vi "Test1.vi"() -> ()   [LabVIEW 2015]
panel:
  out "数值":i32
  in  "停止":bool
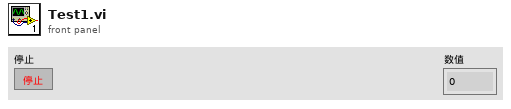
[diagram p1: front panel]
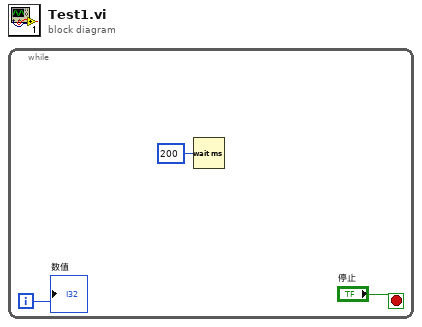
[diagram p0: block diagram]
diagram:
  n1 = while {
    i -> [w1]
    stop <- "停止" stop-if-true
    n2 = Wait (ms)(milliseconds to wait=u32 200 ("等待时间（毫秒）")) -> ()  [unwired: 1 out]
    "数值" <- w1
  }
